vi "Configure List Sweep.vi"(5 "Sweep Function B (0: None)":u16(ring) items=["None", "Impedance Range", "Frequency", "Voltage", "Current", "Bias Voltage", "Bias Current", "DC Source Voltage"], 6 "Sweep Point Array":dbl[](array[numeric])=[0.0, 0.0, 0.0, 0.0, 0.0], 7 "Sweep Function A (0: Frequency)":u16(ring) items=["Frequency", "Voltage", "Current", "Bias Voltage", "Bias Current", "DC Source Voltage"], 8 "error in (no error)":errorcluster, 10 "Sweep Mode (0: Sequence)":u16(ring) items=["Sequence", "Stepped"], 11 "VISA resource name":refnum<visa-resource-name>) -> (0 "error out":errorcluster, 3 "VISA resource name out":refnum<visa-resource-name>)   [LabVIEW 2019, in "Agilent E4980.lvlib"]
doc: "Selects the sweep mode and sweep function. Also sets points values for the selected sweep function."
uses:
  Agilent E4980.lvlib
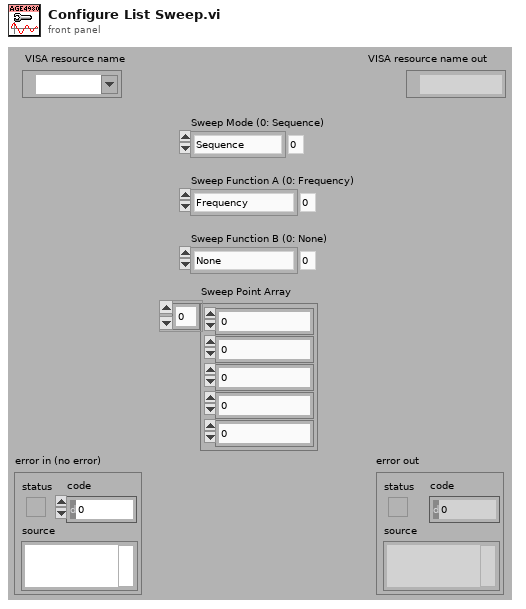
[diagram p1: front panel]
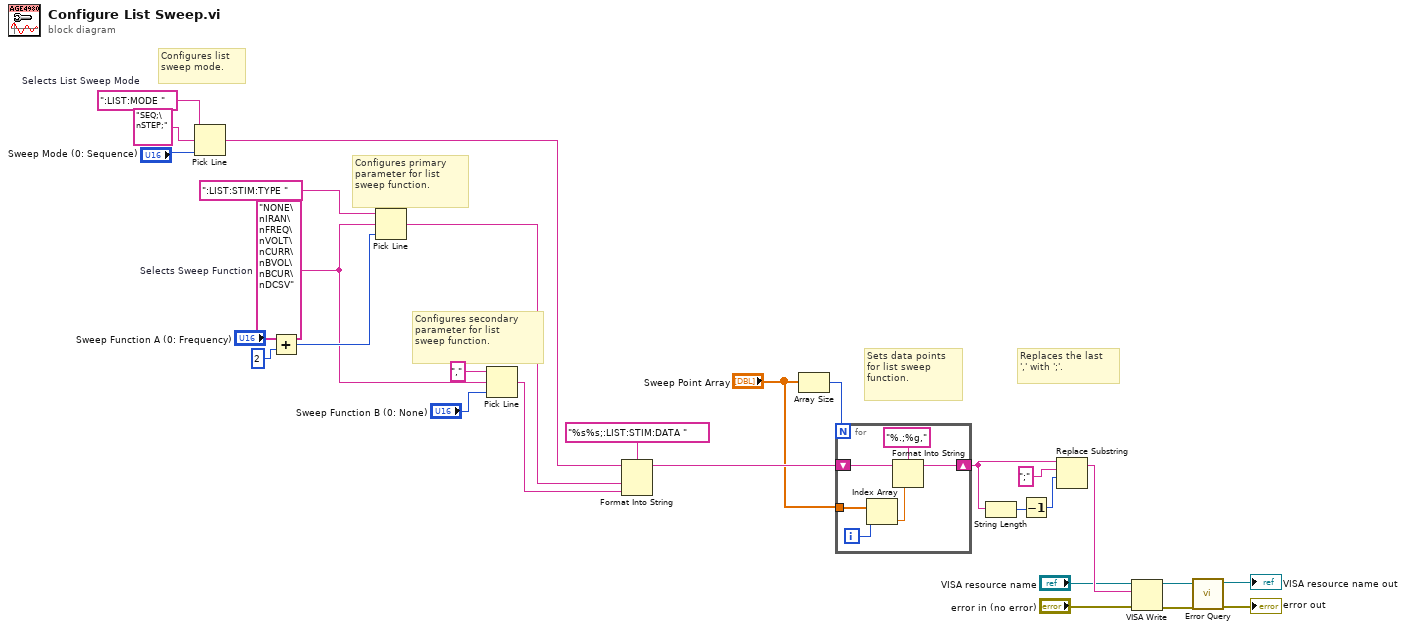
[diagram p0: block diagram]
diagram:
  w20 = "NONE\nIRAN\nFREQ\nVOLT\nCURR\nBVOL\nBCUR\nDCSV"  # Selects Sweep Function
  w26 = ":LIST:MODE "  # Selects List Sweep Mode
  # "Replaces the last\n',' with ';'."
  # "Sets data points\nfor list sweep\nfunction."
  # "Configures secondary\nparameter for list\nsweep function."
  # "Configures primary\nparameter for list\nsweep function."
  # "Configures list\nsweep mode."
  n1 = Pick Line(string ("")=w26, multi-line string="SEQ;\nSTEP;", line index="Sweep Mode (0: Sequence)") -> (output string=w7:string)
  n2 = Add(x="Sweep Function A (0: Frequency)", y=u16 2) -> (x+y=w23:u16)
  n3 = Pick Line(string ("")=":LIST:STIM:TYPE " ("input 1"), multi-line string=w20, line index=w23) -> (output string=w6:string)
  n4 = Pick Line(string ("")=",", multi-line string=w20, line index="Sweep Function B (0: None)") -> (output string=w5:string)
  n5 = Format Into String(format string="%s%s;:LIST:STIM:DATA ", initial string=w7, w6, w5) -> (resulting string=w18:string)  [unwired: 1 in, 1 out]
  n6 = Array Size(array="Sweep Point Array") -> (size(s)=w4:i32)
  n7 = for {
    N: w4 -> [_]
    shift-right: [w32] -> w16
    shift-left: w18 -> [w33]
    tunnel: "Sweep Point Array" -> [w31]
    i -> [w30]
    n8 = Index Array(array=w31, index=w30) -> (element=w29:dbl)
    n9 = Format Into String(format string="%.;%g,", initial string=w33, w29) -> (resulting string=w32:string)  [unwired: 1 in, 1 out]
  }
  n10 = String Length(string=w16) -> (length=w15:i32)
  n11 = Decrement(x=w15) -> (x-1=w9:i32)
  n12 = Replace Substring(3:w9, 4:";" ("substring (\"\")"), 5:w16) -> (1:w3:string)  [unwired: 1 in, 1 out]
  n13 = VISA Write(VISA resource name="VISA resource name", write buffer=w3, error in (no error)="error in (no error)") -> (VISA resource name out=w13:refnum<visa-resource-name>, error out=w12:errorcluster)  [unwired: 1 out]
  n14 = call "Error Query.vi"("error in (no error)"=w12, "VISA resource name"=w13) -> ("error out"=→"error out":errorcluster, "VISA resource name out"=→"VISA resource name out":refnum<visa-resource-name>)  [unwired: 6 in, 2 out]
